vi "SL TAGS Tags to Values.vi"(8 "error in (no error)":errorcluster, 9 "Tag Type":T6, 11 "Tags":T1[](array[typedef])) -> (0 "error out":errorcluster, 3 "Tag Values":T9[](array[typedef]))   [LabVIEW 2017, in "EEISysLink.lvclass"]
doc: "Input a list of tags and return a list of tag values that match a tag type. \n\nJames Tillett P.E.\nEndeavor Engineering Inc.\nwww.endeavoreng.com"
uses:
  EEISysLink.lvclass
  Controls/SL Tag Value.ctl
  Controls/SL Tag Data Type.ctl
  Controls/SL Tag Type.ctl
  Controls/SL Tag.ctl
  <vilib>/Skyline/Tag/Wrapper/Wrapper_class/NI Skyline Tag.lvclass
  Controls/SL Tag Properties.ctl
  Controls/SL Tag Interpolation Method.ctl
  Controls/SL Tag Unit of Measure.ctl
  <vilib>/Skyline/Tag/Shared/typedefs/Tag Cluster.ctl
  <vilib>/Skyline/Tag/Shared/typedefs/DataType.ctl
  <vilib>/Skyline/Tag/Shared/NI Skyline Tag.lvlib
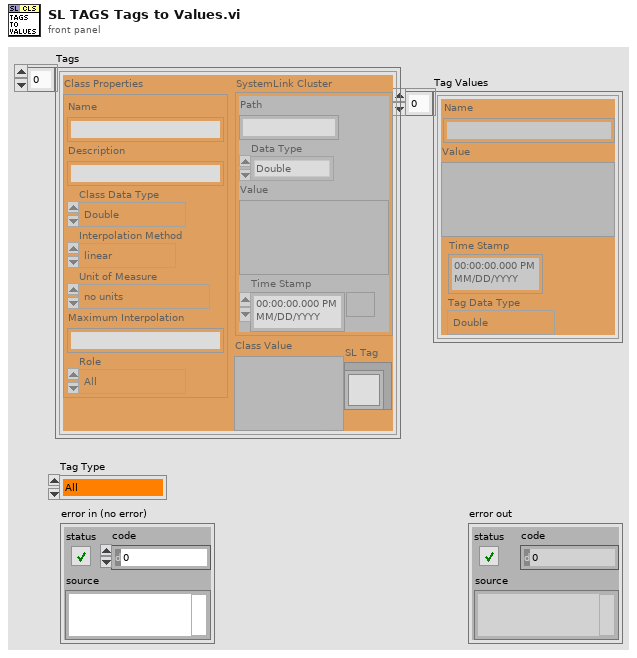
[diagram p1: front panel]
types:
  T1 = typedef "EEISysLink.lvclass/SL Tag.ctl" = cluster{"Class Properties":T2, "SL Tag":refnum<class "NI Skyline Tag.lvclass">, "SystemLink Cluster":T7, "Class Value":variant}
  T2 = typedef "EEISysLink.lvclass/SL Tag Properties.ctl" = cluster{"Class Data Type":T3, "Name":string, "Description":string, "Interpolation Method":T4, "Unit of Measure":T5, "Maximum Interpolation":string, "Role":T6}
  T3 = typedef "EEISysLink.lvclass/SL Tag Data Type.ctl" = enum16{"Double", "Integer", "String", "Boolean", "Waveform"}
  T4 = typedef "EEISysLink.lvclass/SL Tag Interpolation Method.ctl" = enum16{"linear", "pilinear", "step"}
  T5 = typedef "EEISysLink.lvclass/SL Tag Unit of Measure.ctl" = enum16{"no units", "Second", "Hour", "Minute", "Day", "Year", "Month", "Week", "Foot", "Yard", "Meter", "Centimeter", "Inch", "Mile", "Nautical Mile", "Miles per Hour", "Meters per second", "Square meter", "Cubic meter", "Cubic centimeter", "Cubic inch", "Liter", "Gallon", "Gallons dry US", "Gallon UK", "Percent", "Revolutions per minute", "Revolution", "Degree angle", "Astronomical Unit", "Atom", "Atomic mass", "Bar", "Byte", "C (speed of light)", "Curie", "Decibel", "Electron Volt", "Ounce", "Knot", "G", "Grade", "Are", "Hectare", "Faraday", "Franklin", "Gilbert", "Erg", "Lambert", "Maxwell", "Gauss", "Electron mass", "Kilogram force", "Pound force", "Rad", "Centiradian", "Sphere", "Mach", "Fluid Ounces", "Fluid Ounces UK", "Fahrenheit", "Celsius", "Kelvin", "Rankine", "Gram", "Kilogram", "Pound", "Short/US Ton", "Long/UK ton", "Metric ton", "Mole", "Pounds per square inch", "Inches water column", "Torr", "Millitorr", "Millimeter mercury", "Inches mercury", "Bar (2)", "Atmosphere", "Pascal", "Watt", "kiloWatt", "Horsepower", "Kilowatt Hour", "British thermal units", "Millions of BTU", "Ampere", "Candela", "Radian", "Steradian", "Bit", "Hertz", "Newton", "Joule", "Coulomb", "Volt", "Farad", "Ohm", "Siemens", "Weber", "Tesla", "Henry", "Lumen", "Lux", "Becqueral", "Gray", "Sievert", "Katal", "Angstrom", "Light Year", "Parsec", "Point", "Pixel", "Dyne", "Kilogram force (2)", "Pound force (2)", "Rem", "Rutherford", "Roentgen"}
  T6 = typedef "EEISysLink.lvclass/SL Tag Type.ctl" = enum16{"All", "Supervisor", "Worker"}
  T7 = typedef "NI Skyline Tag.lvlib/Tag Cluster.ctl" = cluster{"Path":string, "Data Type":T8, "Value":variant, "Time Stamp":timestamp}
  T8 = typedef "NI Skyline Tag.lvlib/DataType.ctl" = enum32{"Double", "Integer", "String"}
  T9 = typedef "SL Tag Value.ctl" = cluster{"Value":variant, "Time Stamp":timestamp, "Tag Data Type":T3, "Name":string}
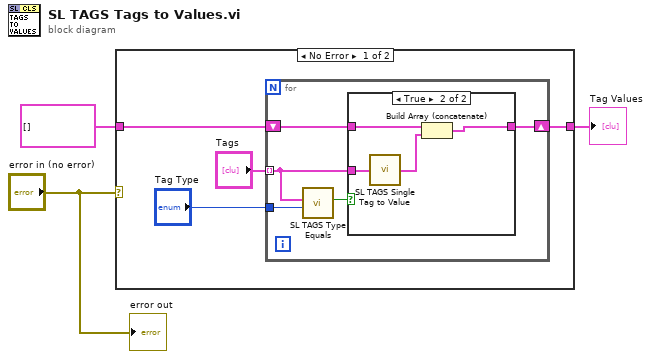
[diagram p0: block diagram]
diagram:
  n1 = case shown="No Error" "error in (no error)" {
    tunnel: [w7 w18] -> w3
    tunnel: T9[] [] -> [w5 w18]
    frame No Error {
      n2 = for {
        tunnel: "Tags" -> [w10] mode=indexing
        shift-right: [w11] -> w7
        shift-left: w5 -> [w12]
        tunnel: "Tag Type" -> [w9]
        n3 = call "SL TAGS Type Equals.vi"("Tag Type"=w9, "Tag"=w10) -> ("Match?"=w8:bool)  [unwired: 9 in]
        n4 = case shown="True" w8 {
          tunnel: w10 -> [_ w15]
          tunnel: w12 -> [w13 w17]
          tunnel: [w13 w16] -> w11
          frame False {
            # "Type doesn't match \nso don't include"
          }
          frame True {
            n5 = call "SL TAGS Single Tag to Value.vi"("Tag"=w15) -> ("Tag Value"=w14:T9)  [unwired: 4 in]
            n6 = Build Array (concatenate)(w17, w14) -> (w16:T9[])
          }
        }
      }
    }
    frame Error {
    }
  }
  "Tag Values" <- w3
  "error out" <- "error in (no error)"
